vi "ief_get_status_all_axis.vi"(0 "Tagprefix in":refnum<k21>, 1 "error in (no error)":errorcluster) -> (2 "Tagprefix out":refnum<k21>, 3 "All Axis State":u16, 4 "error out (no error)":errorcluster)   [LabVIEW 2015, in "IEF Werner.lvlib"]
doc: "The VI returns the present state of all axes.\n\nBit 0 = Axis 1\nBit 1 = Axis 2\n...\nBit 15 = Axis 16\n\nBit State:\nBit = 0 - Axis stopped, in position\nBit = 1 - Axis running\n\nAll Axis State Range:\n0000 - FFFF, hex\n0 - 65535, dec"
uses:
  IEF Werner.lvlib
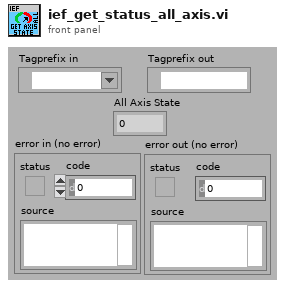
[diagram p1: front panel]
types:
  T1 = typedef "Semaphore RefNum" = refnum<k1>
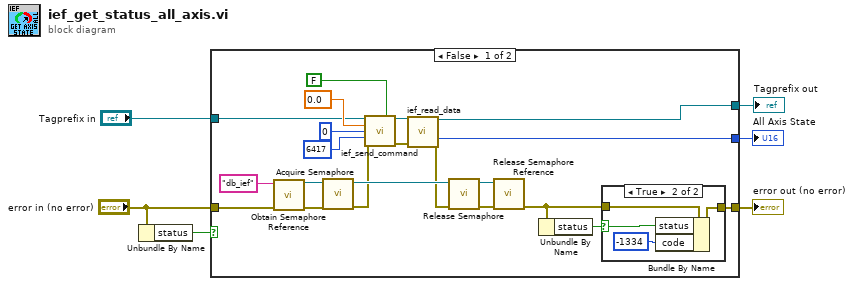
[diagram p0: block diagram]
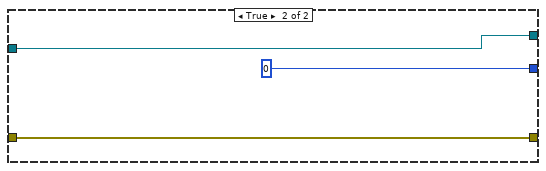
[diagram p3: hidden frame]
diagram:
  n1 = Unbundle By Name("error in (no error)") -> ("status"=w4:bool)
  n2 = case shown="False" w4 {
    tunnel: "error in (no error)" -> [w17 w35]
    tunnel: [w24 w35] -> w6
    tunnel: [w13 u16 0 ("value uint 16")] -> w3
    tunnel: "Tagprefix in" -> [w9 w34]
    tunnel: [w7 w34] -> w1
    frame False {
      n3 = call <vilib>:"Obtain Semaphore Reference.vi"("error in (no error)"=w17, "name (unnamed)"="db_ief") -> ("error out"=w21:errorcluster, "semaphore"=w22:T1)  [unwired: 3 in, 1 out]
      n4 = call <vilib>:"Acquire Semaphore.vi"("error in (no error)"=w21, "semaphore"=w22) -> ("error out"=w16:errorcluster, "semaphore out"=w20:T1)  [unwired: 3 in, 1 out]
      n5 = call "ief_send_command.vi"("Tagprefix in"=w9, "Command datum of type real"=FALSE, "Command datum"=sgl 0.0, "Command parameter"=u16 0, "Command code"=u16 6417, "error in (no error)"=w16) -> ("Tagprefix out"=w8:refnum<k21>, "error out (no error)"=w25:errorcluster)  [unwired: 4 in, 4 out]
      n6 = call "ief_read_data.vi"("Tagprefix in"=w8, "error in (no error)"=w25) -> ("Tagprefix out"=w7:refnum<k21>, "value uint 16"=w13:u16, "error out (no error)"=w15:errorcluster)  [unwired: 7 in, 4 out]
      n7 = call <vilib>:"Release Semaphore.vi"("error in (no error)"=w15, "semaphore"=w20) -> ("error out"=w19:errorcluster, "semaphore out"=w18:T1)  [unwired: 4 in]
      n8 = call <vilib>:"Release Semaphore Reference.vi"("error in (no error)"=w19, "semaphore"=w18) -> ("error out"=w14:errorcluster)  [unwired: 8 in, 1 out]
      n9 = Unbundle By Name(w14) -> ("status"=w12:bool)
      n10 = case shown="True" w12 {
        selector: w12 -> [_ w29]
        tunnel: [w28 w31] -> w24
        tunnel: w14 -> [w28 w32]
        frame False {
        }
        frame True {
          n11 = Bundle By Name(cluster=w32, "status"=w29, "code"=-1334) -> (w31:errorcluster)
        }
      }
    }
    frame True {
    }
  }
  "error out (no error)" <- w6
  "All Axis State" <- w3
  "Tagprefix out" <- w1
